vi "FrontPanel.vi"() -> ()   [LabVIEW 2017, in "AODControl.lvlib"]
uses:
  AODControl.lvlib
  LoadControl.ctl
  InterfaceReferences.ctl
  ExitButton.ctl
  AODSettings.ctl
  AODPointDefinition.ctl
  ListOfPoints.ctl
  <vilib>/Utility/error.llb/DialogType.ctl
  DecodifyFrequency(Array).vi
  MessageQueue/QueueOperations/Enqueue Message (Array).vi
  AODGlobals.vi
  MessageQueue/QueueOperations/Enqueue Message (Single).vi
  MovePoint.vi
  AddPoint.vi
  RemovePoint.vi
  ReplaceList.vi
  AddPoints.vi
  <vilib>/Utility/file.llb/Write To Spreadsheet File (DBL).vi
  <vilib>/Utility/file.llb/Read From Spreadsheet File (DBL).vi
  CodifyFrequency(Array).vi
  MessageQueue/MessageQueue.lvlib
panel:
  in  "Reset Sequence":bool
  out "Sequence":dbl[][][](array[numeric])
  in  "Frame":i32 max=10 step=1
  out "Frames":i32 step=1
  in  "SaveFrame":bool
  in  "Play":bool
  in  "Playing Time":dbl step=0.1
  in  "Tasks":T1={"XTask"="Frequency1", "YTask"="Frequency2"}
  out "Dynamic":bool
  in  "Speed Y":dbl
  in  "Speed Scale":dbl step=0.1
  in  "Speed X":dbl
  in  "Speed Rotate":dbl step=0.1
  in  "Rotate":bool
  in  "Exit Button":T2
  in  "?":T3
  in  "Save List":bool
  in  "Load List":T4
  in  "New List":dbl[][](array[numeric])
  in  "ReplaceList":bool
  out "Number Of Points":i32
  out "Points":dbl[][](array[numeric])
  in  "Add":bool
  out "Display":cluster{dbl[], dbl[]}(graph)
  in  "Move":bool
  in  "Index":i32 min=0 max=81
  in  "Remove":bool
  in  "Y":dbl
  in  "X":dbl
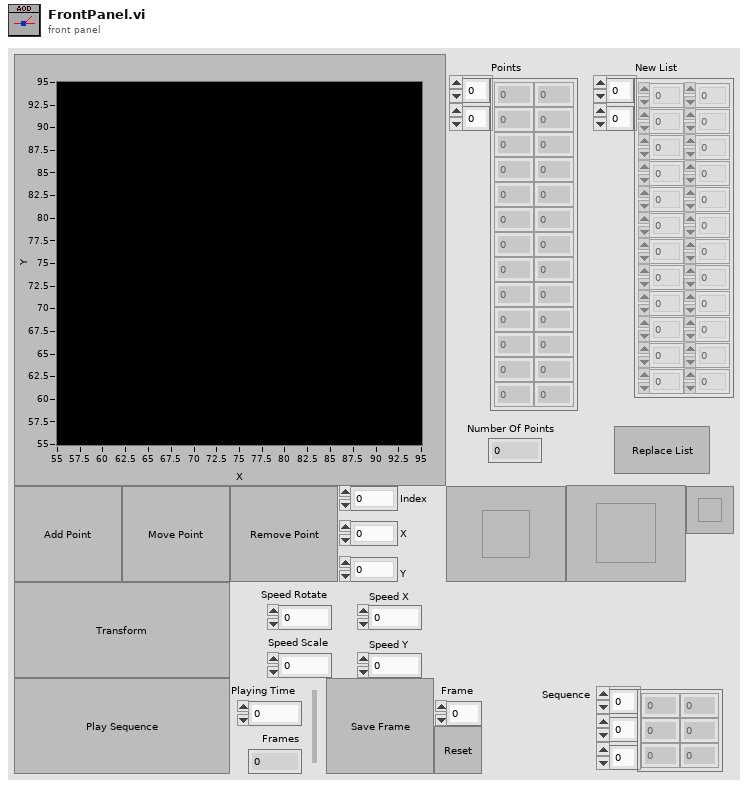
[diagram p1: front panel]
types:
  T1 = typedef "AODControl.lvlib/AODSettings.ctl" = cluster{"XTask":refnum<k21>, "YTask":refnum<k21>}
  T2 = typedef "AODControl.lvlib/ExitButton.ctl" = bool
  T3 = typedef "AODControl.lvlib/InterfaceReferences.ctl" = cluster{"AOD Points Display":refnum<vi>, "AOD Array":refnum<vi>, "AOD Array Size":refnum<vi>, "Replace Array List":refnum<vi>, "Replace List":refnum<vi>, "Remove":refnum<vi>, "Index":refnum<vi>, "Move":refnum<vi>, "X":refnum<vi>, "Y":refnum<vi>, "Add":refnum<vi>, "Load":refnum<vi>, "Save":refnum<vi>, "Exit":refnum<vi>, "Dynamic":refnum<vi>, "Rotate":refnum<vi>, "Rotation Speed":refnum<vi>, "Scaling Speed":refnum<vi>, "X Trans Speed":refnum<vi>, "Y Trans Speed":refnum<vi>, "Movie Array":refnum<vi>, "Play":refnum<vi>, "Playing Time":refnum<vi>}
  T4 = typedef "AODControl.lvlib/LoadControl.ctl" = bool
  T5 = typedef "AODControl.lvlib/ListOfPoints.ctl" = cluster{"X":u32[], "Y":u32[], "Amp":dbl[]}
  T6 = typedef "AODControl.lvlib/AODPointDefinition.ctl" = cluster{"Freq X":dbl, "Freq Y":dbl, "Index":i32, "Ampitude":dbl}
  T7 = typedef "AODControl.lvlib/MessageQueue.lvlib/All Message Queues.ctl" = cluster{" AOD Interface":refnum<queue>}
  T8 = typedef "DialogType.ctl" = u16
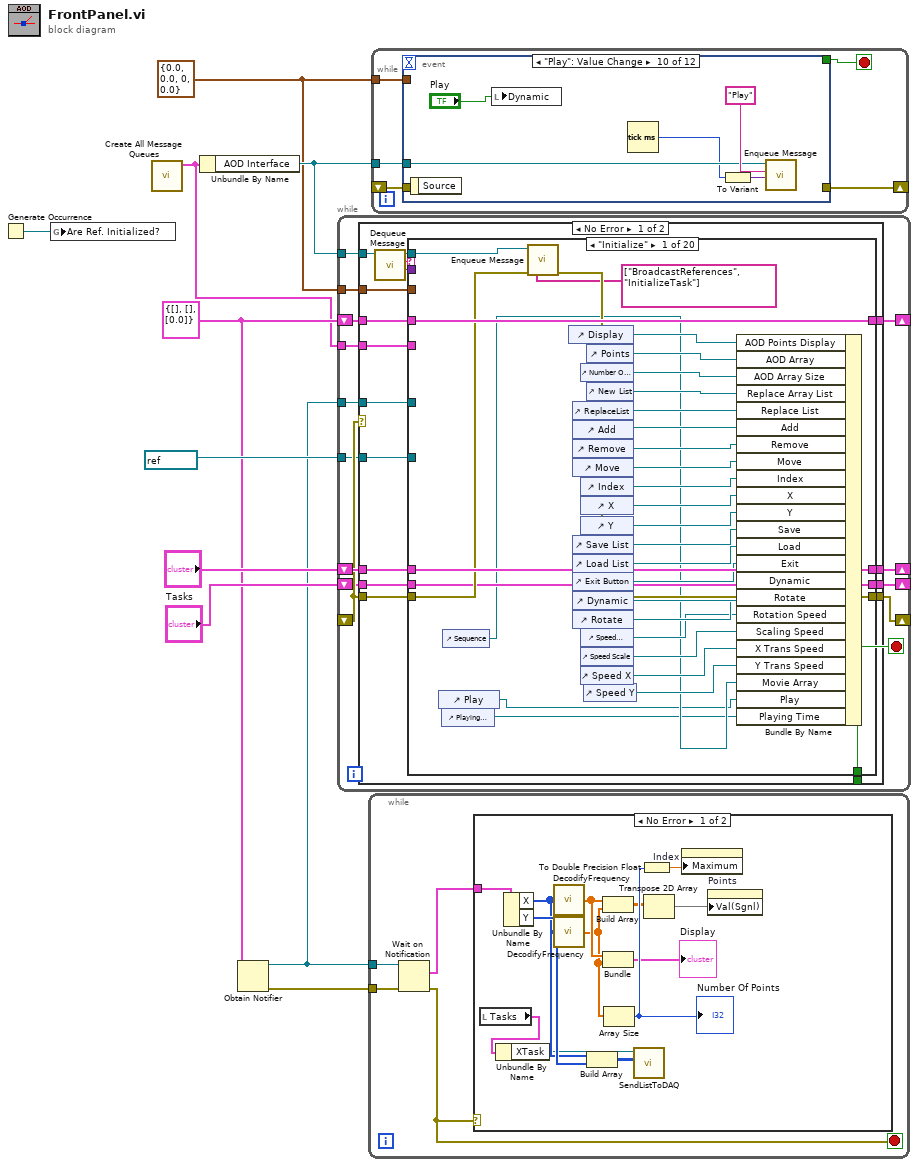
[diagram p0: block diagram]
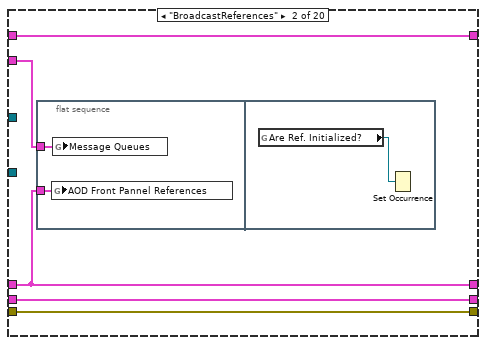
[diagram p3: hidden frame]
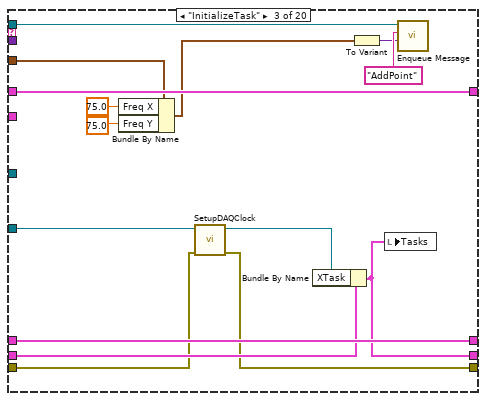
[diagram p4: hidden frame]
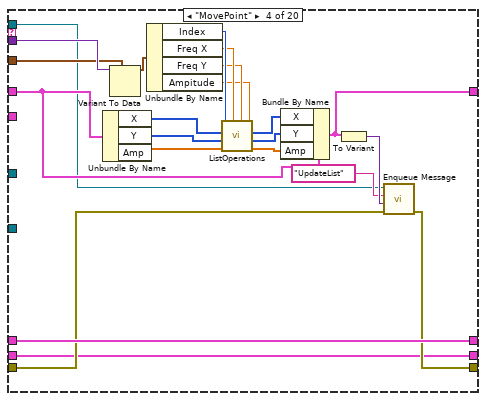
[diagram p5: hidden frame]
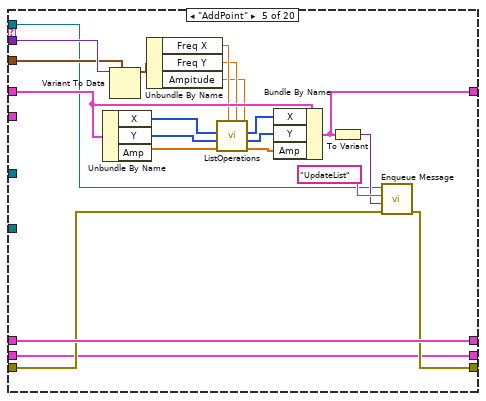
[diagram p6: hidden frame]
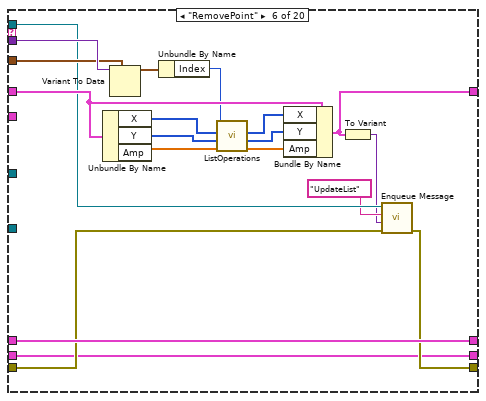
[diagram p7: hidden frame]
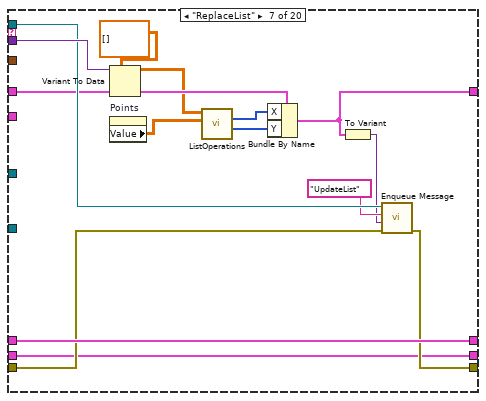
[diagram p8: hidden frame]
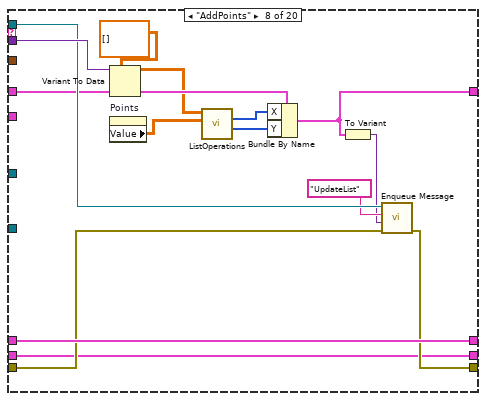
[diagram p9: hidden frame]
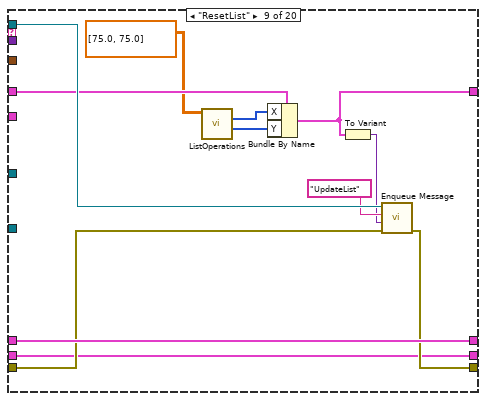
[diagram p10: hidden frame]
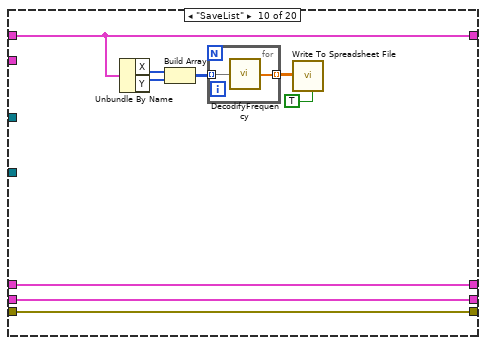
[diagram p11: hidden frame]
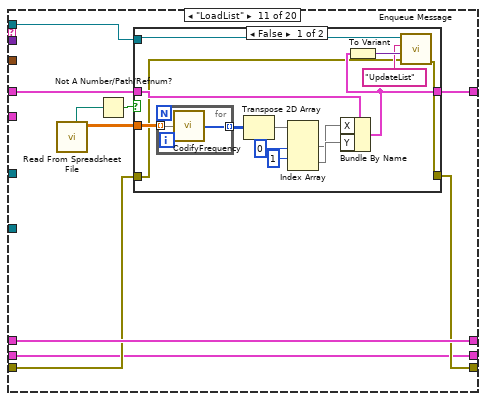
[diagram p12: hidden frame]
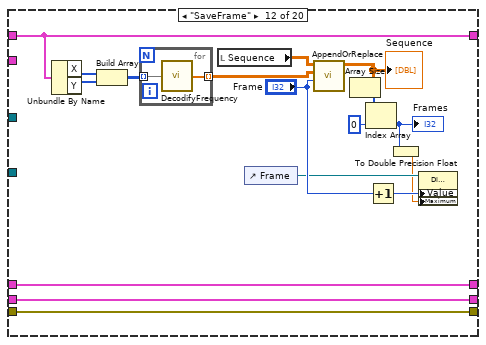
[diagram p14: hidden frame]
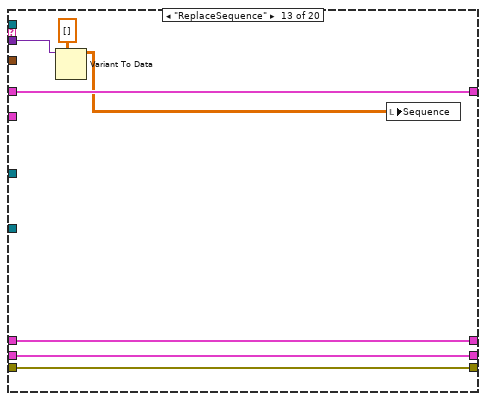
[diagram p15: hidden frame]
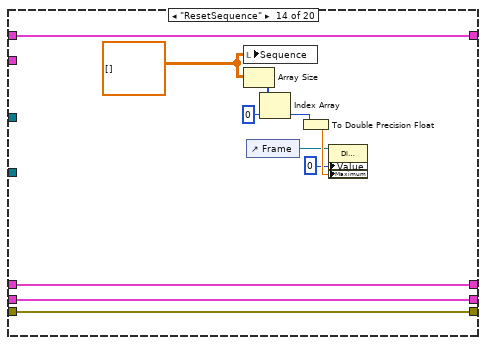
[diagram p16: hidden frame]
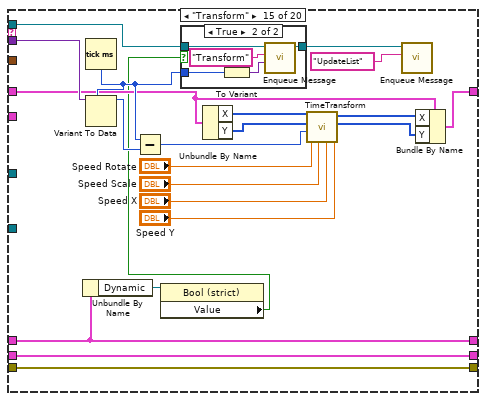
[diagram p17: hidden frame]
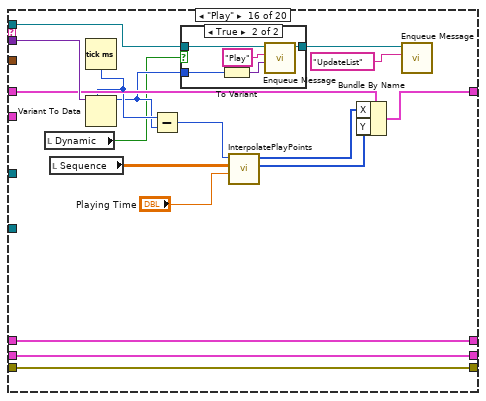
[diagram p19: hidden frame]
diagram:
  w5 = T5 {"X"=[], "Y"=[], "Amp"=[0.0]} ("Cluster")
  w9 = T6 {"Freq X"=0.0, "Freq Y"=0.0, "Index"=0, "Ampitude"=0.0}
  n1 = Generate Occurrence() -> (w1:refnum<k4>)
  n2 = global write "AODGlobals.vi" "Are Ref. Initialized?"(w1) -> ()
  n3 = call "Create All Message Queues.vi"() -> ("Message Queues out"=w2:T7)  [unwired: 10 in, 1 out]
  n4 = Unbundle By Name(w2) -> ("AOD Interface"=w10:refnum<queue>)
  n5 = Obtain Notifier(notification data type=w5) -> (notifier out=w3:refnum<notifier>, error out=w4:errorcluster)  [unwired: 2 in, 2 out]
  n6 = while {
    tunnel: w10 -> [w13]
    shift-right: [w23] -> _
    shift-left: w5 -> [w24]
    tunnel: w9 -> [w21]
    shift-right: [w19] -> _
    shift-left: "?" -> [w20]
    shift-right: [w18] -> _
    shift-left: _ -> [w17]
    shift-right: [w15] -> _
    shift-left: "Tasks" -> [w16]
    tunnel: refnum<k21> "AOD" ("task/channels in") -> [w14]
    tunnel: w3 -> [w12]
    tunnel: w2 -> [w11]
    stop <- w22 stop-if-true
    n7 = case shown="No Error" w17 {
      tunnel: w13 -> [w30 _]
      tunnel: w24 -> [w41 w351]
      tunnel: [w40 w351] -> w23
      tunnel: [w39 _] -> w22
      tunnel: w21 -> [w38 _]
      tunnel: w20 -> [w37 w352]
      tunnel: [w36 w352] -> w19
      tunnel: [w35 w353] -> w18
      tunnel: w17 -> [w34 w354]
      tunnel: w16 -> [w31 w350]
      tunnel: [w33 w350] -> w15
      tunnel: w14 -> [w32 _]
      tunnel: w12 -> [w26 _]
      tunnel: w11 -> [w25 _]
      frame No Error {
        n8 = call "Dequeue Message.vi"("Message Queue"=w30) -> ("Message Data"=w28:variant, "Message"=w27:string, "dup Message Queue"=w29:refnum<queue>)  [unwired: 7 in, 1 out]
        n9 = case shown="\"Initialize\"" w27 {
          tunnel: w29 -> [w60 _ w86 w100 w122 w146 w171 w186 w199 _ w219 _ _ _ w295 w318 _ _ _ _]
          tunnel: w28 -> [_ _ _ w117 w138 w157 w172 w187 _ _ _ _ w259 _ w294 w317 _ _ _ _]
          tunnel: w41 -> [w59 w77 w95 w114 w135 w154 w165 w180 w194 w207 w217 w252 w264 w275 w289 w309 w329 w337 w345 w349]
          tunnel: [w59 w77 w95 w101 w123 w144 w164 w179 w193 w207 w216 w252 w264 w275 w288 w308 w329 w337 w345 w349] -> w40
          tunnel: [_ _ _ _ _ _ _ _ _ _ _ _ _ _ _ _ _ _ TRUE _] -> w39
          tunnel: w38 -> [_ _ w85 w116 w137 w156 _ _ _ _ _ _ _ _ _ _ _ _ _ _]
          tunnel: w37 -> [w72 w75 w94 w99 w121 w142 w162 w177 w192 w208 w220 w250 w263 w274 w278 w314 w332 w336 w343 w348]
          tunnel: [w56 w75 w94 w99 w121 w142 w162 w177 w192 w208 w220 w250 w263 w274 w278 w314 w332 w336 w343 w348] -> w36
          tunnel: [w54 w74 w89 w97 w119 w140 w160 w175 w190 w201 w214 w248 w261 w272 w296 w319 w327 w335 w339 w347] -> w35
          tunnel: w34 -> [w55 w74 w90 w98 w120 w141 w161 w176 w191 w201 w215 w248 w261 w272 w296 w319 w328 w335 w340 w347]
          tunnel: [w53 w76 w81 w96 w118 w139 w159 w174 w189 w200 w211 w249 w262 w273 w297 w320 w331 w334 w342 w346] -> w33
          tunnel: w32 -> [_ _ w93 _ _ _ _ _ _ _ _ _ _ _ _ _ _ _ _ _]
          tunnel: w31 -> [w53 w76 w92 w96 w118 w139 w159 w174 w189 w200 w211 w249 w262 w273 w297 w320 w331 w334 w342 w346]
          tunnel: w26 -> [_ _ _ _ _ _ _ _ _ _ _ _ _ _ _ _ w330 _ w338 _]
          tunnel: w25 -> [_ w73 _ _ _ _ _ _ _ _ _ _ _ _ _ _ _ _ _ _]
          frame "Initialize" {
            n10 = control-ref of="Play"() -> (w43:refnum<vi>)
            n11 = control-ref of="Playing Time"() -> (w42:refnum<vi>)
            n12 = control-ref of="Sequence"() -> (w44:refnum<vi>)
            n13 = call-poly "Enqueue Message.vi"("error in (no error)"=w55, "Message Array"=string[] ["BroadcastReferences", "InitializeTask"], "Message Queue"=w60) -> ("error out"=w54:errorcluster)  [unwired: 7 in, 1 out]
            n14 = control-ref of="Display"() -> (w71:refnum<vi>)
            n15 = control-ref of="ReplaceList"() -> (w67:refnum<vi>)
            n16 = control-ref of="Add"() -> (w66:refnum<vi>)
            n17 = control-ref of="Remove"() -> (w65:refnum<vi>)
            n18 = control-ref of="Move"() -> (w64:refnum<vi>)
            n19 = control-ref of="Save List"() -> (w58:refnum<vi>)
            n20 = control-ref of="Load List"() -> (w57:refnum<vi>)
            n21 = control-ref of="Exit Button"() -> (w50:refnum<vi>)
            n22 = control-ref of="Dynamic"() -> (w51:refnum<vi>)
            n23 = control-ref of="Rotate"() -> (w49:refnum<vi>)
            n24 = control-ref of="Number Of Points"() -> (w69:refnum<vi>)
            n25 = control-ref of="Index"() -> (w63:refnum<vi>)
            n26 = control-ref of="X"() -> (w62:refnum<vi>)
            n27 = control-ref of="Y"() -> (w61:refnum<vi>)
            n28 = control-ref of="Speed Rotate"() -> (w48:refnum<vi>)
            n29 = control-ref of="Speed Scale"() -> (w47:refnum<vi>)
            n30 = control-ref of="Speed X"() -> (w46:refnum<vi>)
            n31 = control-ref of="Speed Y"() -> (w45:refnum<vi>)
            n32 = control-ref of="Points"() -> (w70:refnum<vi>)
            n33 = control-ref of="New List"() -> (w68:refnum<vi>)
            n34 = Bundle By Name(cluster=w72, "AOD Points Display"=w71, "AOD Array"=w70, "AOD Array Size"=w69, "Replace Array List"=w68, "Replace List"=w67, "Add"=w66, "Remove"=w65, "Move"=w64, "Index"=w63, "X"=w62, "Y"=w61, "Save"=w58, "Load"=w57, "Exit"=w50, "Dynamic"=w51, "Rotate"=w49, "Rotation Speed"=w48, "Scaling Speed"=w47, "X Trans Speed"=w46, "Y Trans Speed"=w45, "Movie Array"=w44, "Play"=w43, "Playing Time"=w42) -> (w56:T3)
          }
          frame "BroadcastReferences" {
            n35 = flat-sequence {
              tunnel: w75 -> [w79]
              tunnel: w73 -> [w78]
              frame #0 {
                n36 = global write "AODGlobals.vi" "AOD Front Pannel References"(w79) -> ()
                n37 = global write "AODGlobals.vi" "Message Queues"(w78) -> ()
              }
              frame #1 {
                n38 = global read "AODGlobals.vi" "Are Ref. Initialized?"() -> (w80:refnum<k4>)
                n39 = Set Occurrence(w80) -> ()
              }
            }
          }
          frame "InitializeTask" {
            n40 = Bundle By Name(cluster=w85, "Freq X"=75.0, "Freq Y"=75.0 ("Freq X")) -> (w82:T6)
            n41 = call "SetupDAQClock.vi"("error in"=w90, "task/channels in"=w93) -> ("error out"=w89:errorcluster, "task out"=w91:refnum<k21>)  [unwired: 8 in]
            n42 = Bundle By Name(cluster=w92, "XTask"=w91) -> (w81:T1)
            n43 = To Variant(anything=w82) -> (Variant=w87:variant)
            n44 = local write "Tasks"(w81) -> ()
            n45 = call-poly "Enqueue Message.vi"("Message Data"=w87, "Message"="AddPoint", "Message Queue"=w86) -> ()  [unwired: 7 in, 2 out]
          }
          frame "MovePoint" {
            n46 = Unbundle By Name(w114) -> ("X"=w109:u32[], "Y"=w108:u32[], "Amp"=w107:dbl[])
            n47 = Variant To Data(type=w116, Variant=w117) -> (data=w115:T6)  [unwired: 1 in, 1 out]
            n48 = Unbundle By Name(w115) -> ("Index"=w113:i32, "Freq X"=w112:dbl, "Freq Y"=w111:dbl, "Ampitude"=w110:dbl)
            n49 = call-poly "ListOperations.vi"("Ampitude"=w110, "Freq Y"=w111, "Freq X"=w112, "Amp in"=w107, "Y in"=w108, "X in"=w109, "Index"=w113) -> ("Amp out"=w105:dbl[], "Y out"=w104:u32[], "X out"=w106:u32[])  [unwired: 2 in]
            n50 = Bundle By Name(cluster=w114, "X"=w106, "Y"=w104, "Amp"=w105) -> (w101:T5)
            n51 = To Variant(anything=w101) -> (Variant=w103:variant)
            n52 = call-poly "Enqueue Message.vi"("error in (no error)"=w98, "Message Data"=w103, "Message"="UpdateList", "Message Queue"=w100) -> ("error out"=w97:errorcluster)  [unwired: 6 in, 1 out]
          }
          frame "AddPoint" {
            n53 = Unbundle By Name(w135) -> ("X"=w131:u32[], "Y"=w130:u32[], "Amp"=w129:dbl[])
            n54 = Variant To Data(type=w137, Variant=w138) -> (data=w136:T6)  [unwired: 1 in, 1 out]
            n55 = Unbundle By Name(w136) -> ("Freq X"=w134:dbl, "Freq Y"=w133:dbl, "Ampitude"=w132:dbl)
            n56 = call-poly "ListOperations.vi"("Ampitude"=w132, "Freq Y"=w133, "Freq X"=w134, "Amp in"=w129, "Y in"=w130, "X in"=w131) -> ("Amp out"=w126:dbl[], "Y out"=w127:u32[], "X out"=w128:u32[])  [unwired: 3 in]
            n57 = Bundle By Name(cluster=w135, "X"=w128, "Y"=w127, "Amp"=w126) -> (w123:T5)
            n58 = To Variant(anything=w123) -> (Variant=w124:variant)
            n59 = call-poly "Enqueue Message.vi"("error in (no error)"=w120, "Message Data"=w124, "Message"="UpdateList", "Message Queue"=w122) -> ("error out"=w119:errorcluster)  [unwired: 6 in, 1 out]
          }
          frame "RemovePoint" {
            n60 = Unbundle By Name(w154) -> ("X"=w153:u32[], "Y"=w152:u32[], "Amp"=w151:dbl[])
            n61 = Variant To Data(type=w156, Variant=w157) -> (data=w155:T6)  [unwired: 1 in, 1 out]
            n62 = Unbundle By Name(w155) -> ("Index"=w147:i32)
            n63 = call-poly "ListOperations.vi"("Amp in"=w151, "Y in"=w152, "X in"=w153, "Index"=w147) -> ("Amp out"=w148:dbl[], "Y out"=w149:u32[], "X out"=w150:u32[])  [unwired: 5 in]
            n64 = Bundle By Name(cluster=w154, "X"=w150, "Y"=w149, "Amp"=w148) -> (w144:T5)
            n65 = To Variant(anything=w144) -> (Variant=w143:variant)
            n66 = call-poly "Enqueue Message.vi"("error in (no error)"=w141, "Message Data"=w143, "Message"="UpdateList", "Message Queue"=w146) -> ("error out"=w140:errorcluster)  [unwired: 6 in, 1 out]
          }
          frame "ReplaceList" {
            n67 = Variant To Data(type=dbl[][] [] ("New List"), Variant=w172) -> (data=w163:dbl[][])  [unwired: 1 in, 1 out]
            n68 = property on="Points" class="Arr (strict)"() -> ("Value"=w158:dbl[][])  [unwired: 2 in, 2 out]
            n69 = call-poly "ListOperations.vi"("Old List"=w158, "New List"=w163) -> ("Y"=w166:u32[], "X"=w167:u32[])  [unwired: 8 in]
            n70 = Bundle By Name(cluster=w165, "X"=w167, "Y"=w166) -> (w164:T5)
            n71 = To Variant(anything=w164) -> (Variant=w169:variant)
            n72 = call-poly "Enqueue Message.vi"("error in (no error)"=w161, "Message Data"=w169, "Message"="UpdateList", "Message Queue"=w171) -> ("error out"=w160:errorcluster)  [unwired: 6 in, 1 out]
          }
          frame "AddPoints" {
            n73 = Variant To Data(type=dbl[][] [] ("New List"), Variant=w187) -> (data=w178:dbl[][])  [unwired: 1 in, 1 out]
            n74 = property on="Points" class="Arr (strict)"() -> ("Value"=w173:dbl[][])  [unwired: 2 in, 2 out]
            n75 = call-poly "ListOperations.vi"("Old List"=w173, "New List"=w178) -> ("Y"=w181:u32[], "X"=w182:u32[])  [unwired: 8 in]
            n76 = Bundle By Name(cluster=w180, "X"=w182, "Y"=w181) -> (w179:T5)
            n77 = To Variant(anything=w179) -> (Variant=w184:variant)
            n78 = call-poly "Enqueue Message.vi"("error in (no error)"=w176, "Message Data"=w184, "Message"="UpdateList", "Message Queue"=w186) -> ("error out"=w175:errorcluster)  [unwired: 6 in, 1 out]
          }
          frame "ResetList" {
            n79 = call-poly "ListOperations.vi"("New List"=dbl[][] [[75.0, 75.0]]) -> ("Y"=w195:u32[], "X"=w196:u32[])  [unwired: 9 in]
            n80 = Bundle By Name(cluster=w194, "X"=w196, "Y"=w195) -> (w193:T5)
            n81 = To Variant(anything=w193) -> (Variant=w197:variant)
            n82 = call-poly "Enqueue Message.vi"("error in (no error)"=w191, "Message Data"=w197, "Message"="UpdateList", "Message Queue"=w199) -> ("error out"=w190:errorcluster)  [unwired: 6 in, 1 out]
          }
          frame "SaveList" {
            n83 = Unbundle By Name(w207) -> ("X"=w206:u32[], "Y"=w205:u32[])
            n84 = Build Array(w206, w205) -> (w203:u32[][])
            n85 = for {
              tunnel: w203 -> [w210] mode=indexing
              tunnel: [w209] -> w204 mode=indexing
              n86 = call-poly "DecodifyFrequency.vi"("Array 2"=w210) -> ("Array"=w209:dbl[])
            }
            n87 = call-poly <vilib>:"Write To Spreadsheet File.vi"("transpose? (no:F)"=TRUE, "2D data"=w204) -> ()  [unwired: 6 in, 1 out]
          }
          frame "LoadList" {
            n88 = call-poly <vilib>:"Read From Spreadsheet File.vi"() -> ("all rows"=w218:dbl[][], "new file path (Not A Path if cancelled)"=w213:path)  [unwired: 7 in, 3 out]
            n89 = Not A Number/Path/Refnum?(number/path/refnum=w213) -> (NaN/Path/Refnum?=w212:bool)
            n90 = case shown="False" w212 {
              tunnel: w219 -> [w234 _]
              tunnel: w218 -> [w231 _]
              tunnel: w217 -> [w226 w237]
              tunnel: [w223 w237] -> w216
              tunnel: w215 -> [w222 w238]
              tunnel: [w221 w238] -> w214
              frame False {
                n91 = for {
                  tunnel: w231 -> [w236] mode=indexing
                  tunnel: [w235] -> w230 mode=indexing
                  n92 = call-poly "CodifyFrequency.vi"("Array"=w236) -> ("Array 2"=w235:u32[])
                }
                n93 = Transpose 2D Array(2D array=w230) -> (transposed array=w229:u32[][])
                n94 = Index Array(array=w229, index (row) #1=0 ("index (row)"), index (row) #2=1 ("index (row)")) -> (element #1=w224:u32[], element #2=w225:u32[])  [unwired: 2 in]
                n95 = Bundle By Name(cluster=w226, "X"=w224, "Y"=w225) -> (w223:T5)
                n96 = To Variant(anything=w223) -> (Variant=w233:variant)
                n97 = call-poly "Enqueue Message.vi"("error in (no error)"=w222, "Message Data"=w233, "Message"="UpdateList", "Message Queue"=w234) -> ("error out"=w221:errorcluster)  [unwired: 6 in, 1 out]
              }
              frame True {
              }
            }
          }
          frame "SaveFrame" {
            n98 = Unbundle By Name(w252) -> ("X"=w253:u32[], "Y"=w254:u32[])
            n99 = Build Array(w253, w254) -> (w255:u32[][])
            n100 = for {
              tunnel: w255 -> [w257] mode=indexing
              tunnel: [w256] -> w246 mode=indexing
              n101 = call-poly "DecodifyFrequency.vi"("Array 2"=w257) -> ("Array"=w256:dbl[])
            }
            n102 = local read "Sequence"() -> (w247:dbl[][][])
            n103 = control-ref of="Frame"() -> (w242:refnum<vi>)
            n104 = call "AppendOrReplace.vi"("index 2"="Frame", "new element/subarray 2"=w246, "Sequence 2"=w247) -> ("Sequence"=w245:dbl[][][])  [unwired: 8 in]
            "Sequence" <- w245
            n105 = Array Size(array=w245) -> (size(s)=w251:i32[])
            n106 = Index Array(array=w251, index=0) -> (element=w240:i32)
            "Frames" <- w240
            n107 = Increment(x="Frame") -> (x+1=w241:i32)
            n108 = To Double Precision Float(number=w240) -> (double precision float=w239:dbl)
            n109 = property class="DigNum (strict)"(reference=w242, "Value"=w241, "Maximum"=w239) -> ()  [unwired: 1 in, 2 out]
          }
          frame "ReplaceSequence" {
            n110 = Variant To Data(type=dbl[][][] [] ("Sequence"), Variant=w259) -> (data=w258:dbl[][][])  [unwired: 1 in, 1 out]
            n111 = local write "Sequence"(w258) -> ()
          }
          frame "ResetSequence" {
            w265 = dbl[][][] [] ("Sequence")
            n112 = local write "Sequence"(w265) -> ()
            n113 = Array Size(array=w265) -> (size(s)=w268:i32[])
            n114 = control-ref of="Frame"() -> (w266:refnum<vi>)
            n115 = Index Array(array=w268, index=0) -> (element=w270:i32)
            n116 = To Double Precision Float(number=w270) -> (double precision float=w271:dbl)
            n117 = property class="DigNum (strict)"(reference=w266, "Value"=0 ("Frame"), "Maximum"=w271) -> ()  [unwired: 1 in, 2 out]
          }
          frame "Transform" {
            n118 = Unbundle By Name(w278) -> ("Dynamic"=w277:refnum<vi>)
            n119 = Tick Count (ms)() -> (millisecond timer value=w293:u32)
            n120 = Variant To Data(type=w293, Variant=w294) -> (data=w292:u32)  [unwired: 1 in, 1 out]
            n121 = Subtract(x=w293, y=w292) -> (x-y=w279:u32)
            n122 = property class="Bool (strict)"(reference=w277) -> ("Value"=w276:bool)  [unwired: 1 in, 2 out]
            n123 = case shown="True" w276 {
              tunnel: w295 -> [w298 w303]
              tunnel: w293 -> [_ w300]
              tunnel: [w298 w299] -> w291
              frame False {
              }
              frame True {
                n124 = To Variant(anything=w300) -> (Variant=w301:variant)
                n125 = call-poly "Enqueue Message.vi"("Message Data"=w301, "Message"="Transform", "Message Queue"=w303) -> ("dup Message Queue"=w299:refnum<queue>)  [unwired: 7 in, 1 out]
              }
            }
            n126 = Unbundle By Name(w289) -> ("X"=w287:u32[], "Y"=w286:u32[])
            n127 = call "TimeTransform.vi"("Speed Y"="Speed Y", "Speed X"="Speed X", "Speed Scale"="Speed Scale", "Speed Rotate"="Speed Rotate", "Elapsed Time"=w279, "Y"=w286, "X"=w287) -> ("Y out"=w284:u32[], "X out"=w285:u32[])  [unwired: 3 in]
            n128 = call-poly "Enqueue Message.vi"("Message"="UpdateList", "Message Queue"=w291) -> ()  [unwired: 8 in, 2 out]
            n129 = Bundle By Name(cluster=w289, "X"=w285, "Y"=w284) -> (w288:T5)
          }
          frame "Play" {
            n130 = local read "Dynamic"() -> (w305:bool)
            n131 = local read "Sequence"() -> (w304:dbl[][][])
            n132 = Tick Count (ms)() -> (millisecond timer value=w307:u32)
            n133 = Variant To Data(type=w307, Variant=w317) -> (data=w306:u32)  [unwired: 1 in, 1 out]
            n134 = Subtract(x=w307, y=w306) -> (x-y=w313:u32)
            n135 = case shown="True" w305 {
              tunnel: w318 -> [w321 w326]
              tunnel: w306 -> [_ w323]
              tunnel: [w321 w322] -> w316
              frame False {
              }
              frame True {
                n136 = To Variant(anything=w323) -> (Variant=w324:variant)
                n137 = call-poly "Enqueue Message.vi"("Message Data"=w324, "Message"="Play", "Message Queue"=w326) -> ("dup Message Queue"=w322:refnum<queue>)  [unwired: 7 in, 1 out]
              }
            }
            n138 = call "InterpolatePlayPoints.vi"("Total Playing Time (sec)"="Playing Time", "Point List"=w304, "Ellapsed Time (ms)"=w313) -> ("Y"=w310:u32[], "X"=w311:u32[])  [unwired: 7 in]
            n139 = Bundle By Name(cluster=w309, "X"=w311, "Y"=w310) -> (w308:T5)
            n140 = call-poly "Enqueue Message.vi"("Message"="UpdateList", "Message Queue"=w316) -> ()  [unwired: 8 in, 2 out]
          }
          frame "UpdateList" {
            n141 = Send Notification(notification=w329, notifier=w330, error in (no error)=w328) -> (error out=w327:errorcluster)  [unwired: 1 out]
          }
          frame "ExitFromOutside" {
            n142 = property on="Exit Button" class="Bool (strict)"("Val(Sgnl)"=FALSE) -> ()  [unwired: 2 in, 2 out]
          }
          frame "Exit" {
            n143 = Release Notifier(notifier=w338) -> ()  [unwired: 1 in, 4 out]
            n144 = Unbundle By Name(w342) -> ("XTask"=w341:refnum<k21>)
            n145 = call "StopDAQ.vi"("error in"=w340, "Refnum in"=w341) -> ("error out"=w339:errorcluster)  [unwired: 9 in]
          }
          frame Default {
          }
        }
      }
      frame Error {
        w355 = T8 2 items=["no dialog", "OK message", "continue or stop message", "OK message + warnings", "continue/stop + warnings"] ("type of dialog (OK msg:1)")
        n146 = call <vilib>:"Simple Error Handler.vi"("type of dialog (OK msg:1)"=w355, "error in (no error)"=w354) -> ("error out"=w356:errorcluster)  [unwired: 3 in, 4 out]
        n147 = call <vilib>:"Clear Errors.vi"("error in (no error)"=w356) -> ("error out"=w353:errorcluster)  [unwired: 5 in, 1 out]
      }
    }
  }
  n148 = while {
    tunnel: w3 -> [w359]
    tunnel: w4 -> [w357]
    stop <- w360 stop-if-true
    n149 = Wait on Notification(notifier=w359, error in (no error)=w357) -> (notification=w358:T5, error out=w360:errorcluster)  [unwired: 4 out]
    n150 = case shown="No Error" w360 {
      tunnel: w358 -> [w362 _]
      frame No Error {
        n151 = local read "Tasks"() -> (w361:T1)
        n152 = Unbundle By Name(w361) -> ("XTask"=w367:refnum<k21>)
        n153 = Unbundle By Name(w362) -> ("X"=w369:u32[], "Y"=w370:u32[])
        n154 = call-poly "DecodifyFrequency.vi"("Array 2"=w369) -> ("Array"=w372:dbl[])
        n155 = call-poly "DecodifyFrequency.vi"("Array 2"=w370) -> ("Array"=w371:dbl[])
        n156 = Build Array(w369, w370) -> (w368:u32[][])
        n157 = Build Array(w372, w371) -> (w364:dbl[][])
        n158 = Bundle("Array"=w372, "Array"=w371) -> (→"Display":cluster{"Array":dbl[], "Array":dbl[]})  [unwired: 1 in]
        n159 = Array Size(array=w371) -> (size(s)=w366:i32)
        "Number Of Points" <- w366
        n160 = call "SendListToDAQ.vi"("Input"=w368, "Refnum in"=w367) -> ()  [unwired: 8 in, 2 out]
        n161 = To Double Precision Float(number=w366) -> (double precision float=w365:dbl)
        n162 = Transpose 2D Array(2D array=w364) -> (transposed array=w373:dbl[][])
        n163 = property on="Index" class="DigNum (strict)"("Maximum"=w365) -> ()  [unwired: 2 in, 2 out]
        n164 = property on="Points" class="Arr (strict)"("Val(Sgnl)"=w373) -> ()  [unwired: 2 in, 2 out]
      }
      frame Error {
      }
    }
  }
  n165 = while {
    tunnel: w10 -> [w378]
    tunnel: w9 -> [w377]
    shift-right: [w375] -> _
    shift-left: _ -> [w374]
    stop <- w376 stop-if-true
    n166 = event shown="[9] \"Play\": Value Change" {
      selector: _ -> [_ _ _ _ _ _ _ _ _ _ _ _]
      dyn-events: _ -> [_ _ _ _ _ _ _ _ _ _ _ _]
      timeout: _ -> [_ _ _ _ _ _ _ _ _ _ _ _]
      tunnel: [_ _ _ _ _ _ _ _ _ _ TRUE TRUE] -> w376
      tunnel: w378 -> [w387 w397 w405 w411 w415 w419 w421 w425 w431 w436 w441 w446]
      tunnel: w377 -> [w386 w396 w404 _ _ _ _ _ _ _ _ _]
      tunnel: [w379 w388 w398 w406 w412 w416 w422 w426 _ _ w438 w449] -> w375
      tunnel: w374 -> [w380 w389 w399 w407 w413 w417 w423 w427 _ _ w439 w445]
      event "Add": Value Change {
        n167 = event-data() -> ()  [unwired: 1 in, 1 out]
        n168 = Bundle By Name(cluster=w386, "Freq X"="X", "Freq Y"="Y") -> (w385:T6)
        n169 = To Variant(anything=w385) -> (Variant=w384:variant)
        n170 = call-poly "Enqueue Message.vi"("error in (no error)"=w380, "Message Data"=w384, "Message"="AddPoint", "Message Queue"=w387) -> ("error out"=w379:errorcluster)  [unwired: 6 in, 1 out]
      }
      event "Move": Value Change {
        n171 = event-data() -> ()  [unwired: 1 in, 1 out]
        n172 = property on="X" class="DigNum (strict)"() -> ("Value"=w392:dbl)  [unwired: 2 in, 2 out]
        n173 = property on="Y" class="DigNum (strict)"() -> ("Value"=w391:dbl)  [unwired: 2 in, 2 out]
        n174 = property on="Index" class="DigNum (strict)"() -> ("Value"=w390:i32)  [unwired: 2 in, 2 out]
        n175 = Bundle By Name(cluster=w396, "Freq X"=w392, "Freq Y"=w391, "Index"=w390) -> (w395:T6)
        n176 = To Variant(anything=w395) -> (Variant=w394:variant)
        n177 = call-poly "Enqueue Message.vi"("error in (no error)"=w389, "Message Data"=w394, "Message"="MovePoint", "Message Queue"=w397) -> ("error out"=w388:errorcluster)  [unwired: 6 in, 1 out]
      }
      event "Remove": Value Change {
        n178 = event-data() -> ()  [unwired: 1 in, 1 out]
        n179 = Bundle By Name(cluster=w404, "Index"="Index") -> (w403:T6)
        n180 = To Variant(anything=w403) -> (Variant=w402:variant)
        n181 = call-poly "Enqueue Message.vi"("error in (no error)"=w399, "Message Data"=w402, "Message"="RemovePoint", "Message Queue"=w405) -> ("error out"=w398:errorcluster)  [unwired: 6 in, 1 out]
      }
      event "ReplaceList": Value Change {
        n182 = event-data() -> ()  [unwired: 1 in, 1 out]
        n183 = To Variant(anything="New List") -> (Variant=w410:variant)
        n184 = call-poly "Enqueue Message.vi"("error in (no error)"=w407, "Message Data"=w410, "Message"="ReplaceList", "Message Queue"=w411) -> ("error out"=w406:errorcluster)  [unwired: 6 in, 1 out]
      }
      event "Save List": Value Change {
        n185 = event-data() -> ()  [unwired: 1 in, 1 out]
        n186 = call-poly "Enqueue Message.vi"("error in (no error)"=w413, "Message"="SaveList", "Message Queue"=w415) -> ("error out"=w412:errorcluster)  [unwired: 7 in, 1 out]
      }
      event Value Change {
        n187 = event-data() -> ()  [unwired: 1 in, 1 out]
        n188 = call-poly "Enqueue Message.vi"("error in (no error)"=w417, "Message"="LoadList", "Message Queue"=w419) -> ("error out"=w416:errorcluster)  [unwired: 7 in, 1 out]
      }
      event "SaveFrame": Value Change {
        n189 = event-data() -> ()  [unwired: 1 in, 1 out]
        n190 = call-poly "Enqueue Message.vi"("error in (no error)"=w423, "Message"="SaveFrame", "Message Queue"=w421) -> ("error out"=w422:errorcluster)  [unwired: 7 in, 1 out]
      }
      event "Reset Sequence": Value Change {
        n191 = event-data() -> ()  [unwired: 1 in, 1 out]
        n192 = call-poly "Enqueue Message.vi"("error in (no error)"=w427, "Message"="ResetSequence", "Message Queue"=w425) -> ("error out"=w426:errorcluster)  [unwired: 7 in, 1 out]
      }
      event "Rotate": Value Change {
        n193 = event-data() -> ()  [unwired: 1 in, 1 out]
        n194 = Tick Count (ms)() -> (millisecond timer value=w428:u32)
        n195 = To Variant(anything=w428) -> (Variant=w429:variant)
        n196 = call-poly "Enqueue Message.vi"("Message Data"=w429, "Message"="Transform", "Message Queue"=w431) -> ()  [unwired: 7 in, 2 out]
        "Dynamic" <- "Rotate"
      }
      event "Play": Value Change {
        n197 = event-data() -> ()  [unwired: 1 in, 1 out]
        n198 = local write "Dynamic"("Play") -> ()
        n199 = Tick Count (ms)() -> (millisecond timer value=w434:u32)
        n200 = To Variant(anything=w434) -> (Variant=w435:variant)
        n201 = call-poly "Enqueue Message.vi"("Message Data"=w435, "Message"="Play", "Message Queue"=w436) -> ()  [unwired: 7 in, 2 out]
      }
      event Panel Close {
        n202 = event-data() -> ()  [unwired: 1 in, 1 out]
        n203 = call-poly "Enqueue Message.vi"("error in (no error)"=w439, "Message"="Exit", "Message Queue"=w441) -> ("error out"=w438:errorcluster)  [unwired: 7 in, 1 out]
      }
      event Value Change {
        n204 = event-data() -> ()  [unwired: 1 in, 3 out]
        n205 = Flush Queue(queue=w446, error in (no error)=w445) -> (queue out=w443:refnum<queue>, error out=w444:errorcluster)  [unwired: 1 out]
        n206 = control-ref of="Exit Button"() -> (w448:refnum<vi>)
        n207 = call-poly "Enqueue Message.vi"("error in (no error)"=w444, "Message"="Exit", "Message Queue"=w443) -> ("error out"=w449:errorcluster)  [unwired: 7 in, 1 out]
        n208 = property class="Bool (strict)"(reference=w448, "Value"=T2 FALSE) -> ()  [unwired: 1 in, 2 out]
      }
    }
  }
